vi "VI Tree.vi"   [LabVIEW 2016, in "Keithley DMM6500 DAQ6500 Series.lvlib"]
doc: "This is the instrument driver for the Keithley DMM6500 DAQ6500 Seriess. The VI Tree displays all the user-callable VIs of the instrument driver in an organized table."
uses:
  Keithley DMM6500 DAQ6500 Series.lvlib
  Data/Read (Multiple Points).vi
  Data/Low Level/Fetch (Single).vi
  Configure/Configure Temperature (Thermocouple).vi
panel:
  # "(c) 2018 National Instruments.  ALL RIGHTS RESERVED."
  # "SEE DIAGRAM\nFOR VI TREE."
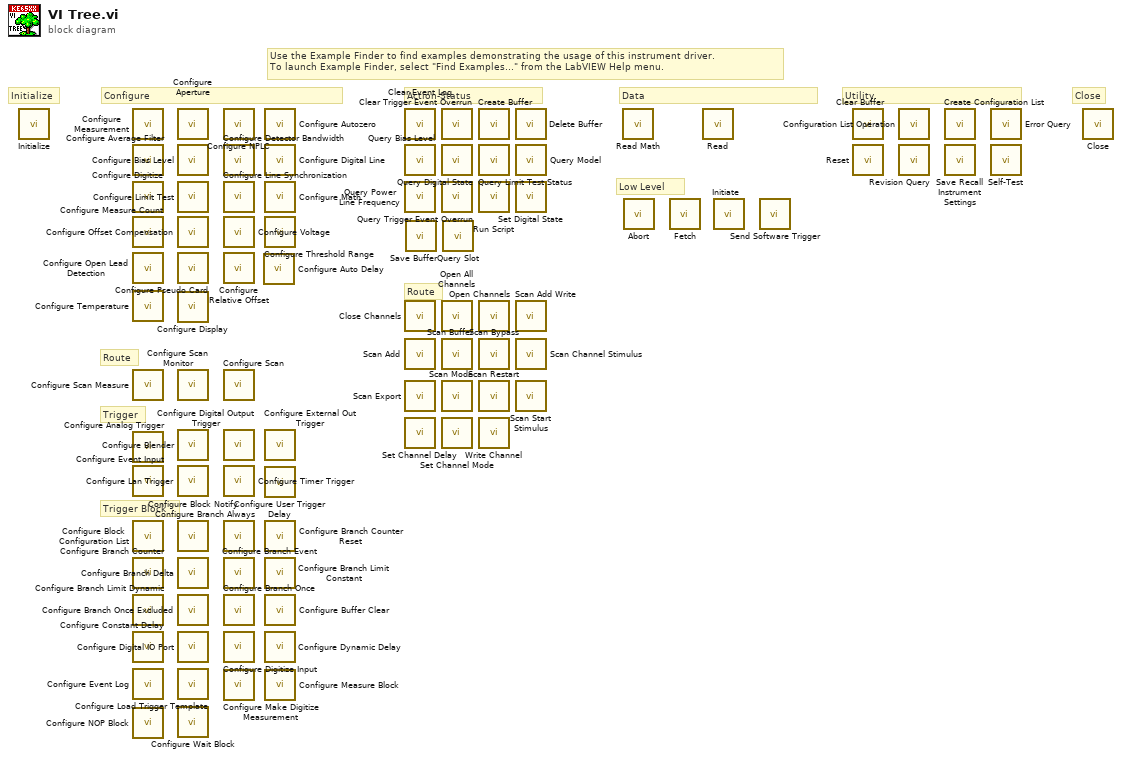
[diagram p0: block diagram]
diagram:
  # "Close"
  # "Utility"
  # "Low Level"
  # "Data"
  # "Trigger Block"
  # "Trigger"
  # "Route"
  # "Configure"
  # "Route"
  # "Action-Status"
  # "Initialize"
  # "Use the Example Finder to find examples demonstrating the usage of this instrument driver.\nTo launch Example Finder, select \"Find Examples...\" from the LabVIEW Help menu."
  n1 = call "Initialize.vi"() -> ()  [unwired: 10 in, 2 out]
  n2 = call "Configure Measurement.vi"() -> ()  [unwired: 10 in, 2 out]
  n3 = call "Configure Average Filter.vi"() -> ()  [unwired: 14 in, 2 out]
  n4 = call "Configure Digitize.vi"() -> ()  [unwired: 10 in, 2 out]
  n5 = call "Configure Measure Count.vi"() -> ()  [unwired: 10 in, 2 out]
  n6 = call "Configure Open Lead Detection.vi"() -> ()  [unwired: 10 in, 2 out]
  n7 = call-poly "Configure Temperature.vi"() -> ()  [unwired: 14 in, 2 out]
  n8 = call "Configure Scan Measure.vi"() -> ()  [unwired: 14 in, 2 out]
  n9 = call "Configure Analog Trigger.vi"() -> ()  [unwired: 14 in, 2 out]
  n10 = call "Configure Event Input.vi"() -> ()  [unwired: 10 in, 2 out]
  n11 = call "Configure Block Configuration List.vi"() -> ()  [unwired: 10 in, 2 out]
  n12 = call "Configure Branch Counter.vi"() -> ()  [unwired: 10 in, 2 out]
  n13 = call "Configure Branch Limit Dynamic.vi"() -> ()  [unwired: 10 in, 2 out]
  n14 = call "Configure Constant Delay.vi"() -> ()  [unwired: 10 in, 2 out]
  n15 = call "Configure Event Log.vi"() -> ()  [unwired: 10 in, 2 out]
  n16 = call "Configure NOP Block.vi"() -> ()  [unwired: 10 in, 2 out]
  n17 = call "Configure Aperture.vi"() -> ()  [unwired: 10 in, 2 out]
  n18 = call "Configure Bias Level.vi"() -> ()  [unwired: 10 in, 2 out]
  n19 = call "Configure Limit Test.vi"() -> ()  [unwired: 14 in, 2 out]
  n20 = call "Configure Offset Compensation.vi"() -> ()  [unwired: 10 in, 2 out]
  n21 = call "Configure Pseudo Card.vi"() -> ()  [unwired: 10 in, 2 out]
  n22 = call "Configure Display.vi"() -> ()  [unwired: 10 in, 2 out]
  n23 = call "Configure Scan Monitor.vi"() -> ()  [unwired: 14 in, 2 out]
  n24 = call "Configure Blender.vi"() -> ()  [unwired: 10 in, 2 out]
  n25 = call "Configure Lan Trigger.vi"() -> ()  [unwired: 10 in, 2 out]
  n26 = call "Configure Block Notify.vi"() -> ()  [unwired: 10 in, 2 out]
  n27 = call "Configure Branch Delta.vi"() -> ()  [unwired: 10 in, 2 out]
  n28 = call "Configure Branch Once Excluded.vi"() -> ()  [unwired: 10 in, 2 out]
  n29 = call "Configure Digital IO Port.vi"() -> ()  [unwired: 10 in, 2 out]
  n30 = call "Configure Load Trigger Template.vi"() -> ()  [unwired: 10 in, 2 out]
  n31 = call "Configure Wait Block.vi"() -> ()  [unwired: 10 in, 2 out]
  n32 = call "Configure NPLC.vi"() -> ()  [unwired: 10 in, 2 out]
  n33 = call "Configure Detector Bandwidth.vi"() -> ()  [unwired: 10 in, 2 out]
  n34 = call "Configure Line Synchronization.vi"() -> ()  [unwired: 10 in, 2 out]
  n35 = call "Configure Voltage.vi"() -> ()  [unwired: 14 in, 2 out]
  n36 = call "Configure Relative Offset.vi"() -> ()  [unwired: 10 in, 2 out]
  n37 = call "Configure Scan.vi"() -> ()  [unwired: 10 in, 2 out]
  n38 = call "Configure Digital Output Trigger.vi"() -> ()  [unwired: 10 in, 2 out]
  n39 = call "Configure Timer Trigger.vi"() -> ()  [unwired: 14 in, 2 out]
  n40 = call "Configure Branch Always.vi"() -> ()  [unwired: 10 in, 2 out]
  n41 = call "Configure Branch Event.vi"() -> ()  [unwired: 10 in, 2 out]
  n42 = call "Configure Branch Once.vi"() -> ()  [unwired: 10 in, 2 out]
  n43 = call "Configure Digitize Input.vi"() -> ()  [unwired: 10 in, 2 out]
  n44 = call "Configure Make Digitize Measurement.vi"() -> ()  [unwired: 10 in, 2 out]
  n45 = call "Configure Auto Delay.vi"() -> ()  [unwired: 10 in, 2 out]
  n46 = call "Configure Autozero.vi"() -> ()  [unwired: 10 in, 2 out]
  n47 = call "Configure Digital Line.vi"() -> ()  [unwired: 10 in, 2 out]
  n48 = call "Configure Math.vi"() -> ()  [unwired: 14 in, 2 out]
  n49 = call "Configure Threshold Range.vi"() -> ()  [unwired: 10 in, 2 out]
  n50 = call "Configure External Out Trigger.vi"() -> ()  [unwired: 10 in, 2 out]
  n51 = call "Configure User Trigger Delay.vi"() -> ()  [unwired: 10 in, 2 out]
  n52 = call "Configure Branch Counter Reset.vi"() -> ()  [unwired: 10 in, 2 out]
  n53 = call "Configure Branch Limit Constant.vi"() -> ()  [unwired: 14 in, 2 out]
  n54 = call "Configure Buffer Clear.vi"() -> ()  [unwired: 10 in, 2 out]
  n55 = call "Configure Dynamic Delay.vi"() -> ()  [unwired: 10 in, 2 out]
  n56 = call "Configure Measure Block.vi"() -> ()  [unwired: 10 in, 2 out]
  n57 = call "Clear Event Log.vi"() -> ()  [unwired: 10 in, 2 out]
  n58 = call "Query Bias Level.vi"() -> ()  [unwired: 9 in, 3 out]
  n59 = call "Query Power Line Frequency.vi"() -> ()  [unwired: 9 in, 3 out]
  n60 = call "Close Channels.vi"() -> ()  [unwired: 10 in, 2 out]
  n61 = call "Scan Add.vi"() -> ()  [unwired: 10 in, 2 out]
  n62 = call "Scan Export.vi"() -> ()  [unwired: 10 in, 2 out]
  n63 = call "Set Channel Delay.vi"() -> ()  [unwired: 10 in, 2 out]
  n64 = call "Save Buffer.vi"() -> ()  [unwired: 10 in, 2 out]
  n65 = call "Clear Trigger Event Overrun.vi"() -> ()  [unwired: 10 in, 2 out]
  n66 = call "Query Digital State.vi"() -> ()  [unwired: 9 in, 3 out]
  n67 = call "Query Trigger Event Overrun.vi"() -> ()  [unwired: 9 in, 3 out]
  n68 = call "Open All Channels.vi"() -> ()  [unwired: 10 in, 2 out]
  n69 = call "Scan Buffer.vi"() -> ()  [unwired: 10 in, 2 out]
  n70 = call "Scan Mode.vi"() -> ()  [unwired: 10 in, 2 out]
  n71 = call "Set Channel Mode.vi"() -> ()  [unwired: 10 in, 2 out]
  n72 = call "Query Slot.vi"() -> ()  [unwired: 9 in, 3 out]
  n73 = call "Create Buffer.vi"() -> ()  [unwired: 10 in, 2 out]
  n74 = call "Query Limit Test Status.vi"() -> ()  [unwired: 8 in, 4 out]
  n75 = call "Run Script.vi"() -> ()  [unwired: 10 in, 2 out]
  n76 = call "Open Channels.vi"() -> ()  [unwired: 10 in, 2 out]
  n77 = call "Scan Bypass.vi"() -> ()  [unwired: 10 in, 2 out]
  n78 = call "Scan Restart.vi"() -> ()  [unwired: 10 in, 2 out]
  n79 = call "Write Channel.vi"() -> ()  [unwired: 10 in, 2 out]
  n80 = call "Delete Buffer.vi"() -> ()  [unwired: 10 in, 2 out]
  n81 = call "Query Model.vi"() -> ()  [unwired: 9 in, 3 out]
  n82 = call "Set Digital State.vi"() -> ()  [unwired: 10 in, 2 out]
  n83 = call "Scan Add Write.vi"() -> ()  [unwired: 10 in, 2 out]
  n84 = call "Scan Channel Stimulus.vi"() -> ()  [unwired: 10 in, 2 out]
  n85 = call "Scan Start Stimulus.vi"() -> ()  [unwired: 10 in, 2 out]
  n86 = call "Read Math.vi"() -> ()  [unwired: 9 in, 7 out]
  n87 = call "Abort.vi"() -> ()  [unwired: 10 in, 2 out]
  n88 = call-poly "Fetch.vi"() -> ()  [unwired: 9 in, 3 out]
  n89 = call-poly "Read.vi"() -> ()  [unwired: 13 in, 3 out]
  n90 = call "Initiate.vi"() -> ()  [unwired: 10 in, 2 out]
  n91 = call "Send Software Trigger.vi"() -> ()  [unwired: 10 in, 2 out]
  n92 = call "Clear Buffer.vi"() -> ()  [unwired: 10 in, 2 out]
  n93 = call "Reset.vi"() -> ()  [unwired: 10 in, 2 out]
  n94 = call "Configuration List Operation.vi"() -> ()  [unwired: 10 in, 2 out]
  n95 = call "Revision Query.vi"() -> ()  [unwired: 8 in, 4 out]
  n96 = call "Create Configuration List.vi"() -> ()  [unwired: 10 in, 2 out]
  n97 = call "Save Recall Instrument Settings.vi"() -> ()  [unwired: 10 in, 2 out]
  n98 = call "Error Query.vi"() -> ()  [unwired: 8 in, 4 out]
  n99 = call "Self-Test.vi"() -> ()  [unwired: 8 in, 4 out]
  n100 = call "Close.vi"() -> ()  [unwired: 11 in, 1 out]
